vi "while.vi"() -> ()   [LabVIEW 2021]
panel:
  out "Numeric":dbl
  out "Tank 2":dbl(slide) scale=0.0..50.0
  in  "Stop":bool
  in  "Vertical Pointer Slide":dbl(slide) scale=0.0..10.0
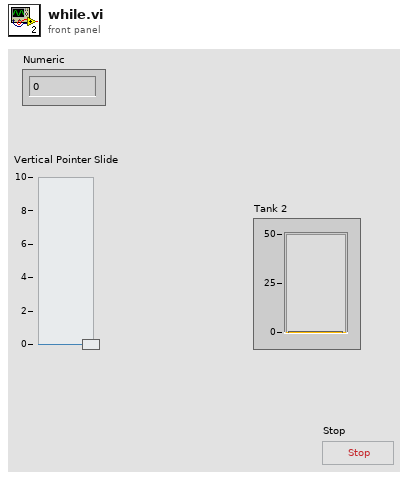
[diagram p1: front panel]
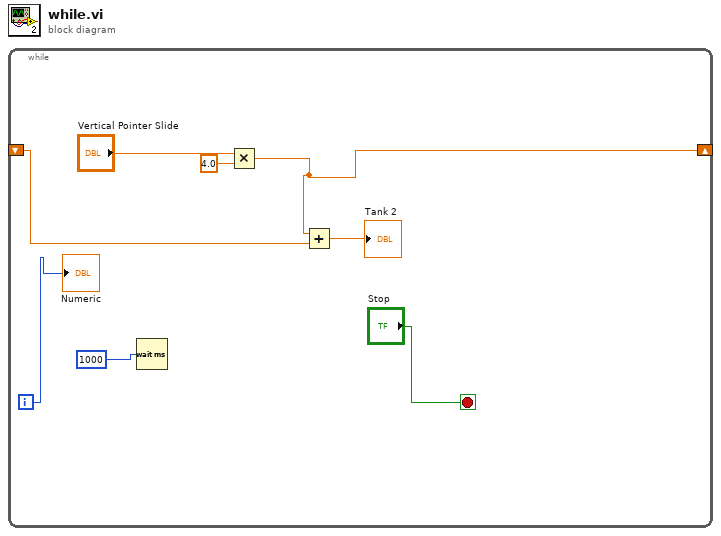
[diagram p0: block diagram]
diagram:
  n1 = while {
    shift-right: [w3] -> _
    shift-left: _ -> [w2]
    i -> [w4]
    stop <- "Stop" stop-if-true
    n2 = Wait (ms)(milliseconds to wait=u32 1000 ("millisecond timer value")) -> ()  [unwired: 1 out]
    n3 = Multiply(x="Vertical Pointer Slide", y=4.0) -> (x*y=w3:dbl)
    n4 = Add(x=w3, y=w2) -> (x+y=→"Tank 2":dbl)
    "Numeric" <- w4
  }
